vi "CAN 6 SPARK MAX Drivetrain Config.vi"() -> (14 "SPARK MAX Ref":T1={"FrontLeftMaster"={"DeviceStatus"={"status"=FALSE, "code"=0, "source"=""}, "Type"=enum."PWM", "PWM"={"PWM Channel"=enum."PWM 1", "DeadBand"={"Name"="", "maxPositivePwm"=0, "minPositivePwm"=0, "centerPwm"=0, "maxNegativePwm"=0, "minNegativePwm"=0, "angularRange"=0}}, "CAN"={"Device Number"=0, "SetOutput VI Ref"=variant(enum8{"Percent VBus", "Current", "Speed", "Position", "Voltage"} enum."Percent VBus"), "GetOutput VI Ref"=variant(refnum<k1> refnum), "Enable VI Ref"=variant(dbl 12.0), "Disable VI Ref"=variant(enum8{"Percent VBus", "Speed", "Position", "Slave", "Unchanged / Invalid", "Voltage Compensation", "Current", "Motion Profile"} enum."Percent VBus"), "Data"=variant}, "Invert"=FALSE, "DIO PWM"={"PWM \"Enable\" Channel"=enum."Invalid", "DIOChannel"=enum."Invalid", "PWM Rate"=0.0}}, "FrontLeftSlave1"={"DeviceStatus"={"status"=FALSE, "code"=0, "source"=""}, "Type"=enum."PWM", "PWM"={"PWM Channel"=enum."PWM 1", "DeadBand"={"Name"="", "maxPositivePwm"=0, "minPositivePwm"=0, "centerPwm"=0, "maxNegativePwm"=0, "minNegativePwm"=0, "angularRange"=0}}, "CAN"={"Device Number"=0, "SetOutput VI Ref"=variant(enum8{"Percent VBus", "Current", "Speed", "Position", "Voltage"} enum."Percent VBus"), "GetOutput VI Ref"=variant(refnum<k1> refnum), "Enable VI Ref"=variant(dbl 12.0), "Disable VI Ref"=variant(enum8{"Percent VBus", "Speed", "Position", "Slave", "Unchanged / Invalid", "Voltage Compensation", "Current", "Motion Profile"} enum."Percent VBus"), "Data"=variant}, "Invert"=FALSE, "DIO PWM"={"PWM \"Enable\" Channel"=enum."Invalid", "DIOChannel"=enum."Invalid", "PWM Rate"=0.0}}, "FrontLeftSlave2"={"DeviceStatus"={"status"=FALSE, "code"=0, "source"=""}, "Type"=enum."PWM", "PWM"={"PWM Channel"=enum."PWM 1", "DeadBand"={"Name"="", "maxPositivePwm"=0, "minPositivePwm"=0, "centerPwm"=0, "maxNegativePwm"=0, "minNegativePwm"=0, "angularRange"=0}}, "CAN"={"Device Number"=0, "SetOutput VI Ref"=variant(enum8{"Percent VBus", "Current", "Speed", "Position", "Voltage"} enum."Percent VBus"), "GetOutput VI Ref"=variant(refnum<k1> refnum), "Enable VI Ref"=variant(dbl 12.0), "Disable VI Ref"=variant(enum8{"Percent VBus", "Speed", "Position", "Slave", "Unchanged / Invalid", "Voltage Compensation", "Current", "Motion Profile"} enum."Percent VBus"), "Data"=variant}, "Invert"=FALSE, "DIO PWM"={"PWM \"Enable\" Channel"=enum."Invalid", "DIOChannel"=enum."Invalid", "PWM Rate"=0.0}}, "FrontRightMaster"={"DeviceStatus"={"status"=FALSE, "code"=0, "source"=""}, "Type"=enum."PWM", "PWM"={"PWM Channel"=enum."PWM 1", "DeadBand"={"Name"="", "maxPositivePwm"=0, "minPositivePwm"=0, "centerPwm"=0, "maxNegativePwm"=0, "minNegativePwm"=0, "angularRange"=0}}, "CAN"={"Device Number"=0, "SetOutput VI Ref"=variant(enum8{"Percent VBus", "Current", "Speed", "Position", "Voltage"} enum."Percent VBus"), "GetOutput VI Ref"=variant(refnum<k1> refnum), "Enable VI Ref"=variant(dbl 12.0), "Disable VI Ref"=variant(enum8{"Percent VBus", "Speed", "Position", "Slave", "Unchanged / Invalid", "Voltage Compensation", "Current", "Motion Profile"} enum."Percent VBus"), "Data"=variant}, "Invert"=FALSE, "DIO PWM"={"PWM \"Enable\" Channel"=enum."Invalid", "DIOChannel"=enum."Invalid", "PWM Rate"=0.0}}, "FrontRightSlave1"={"DeviceStatus"={"status"=FALSE, "code"=0, "source"=""}, "Type"=enum."PWM", "PWM"={"PWM Channel"=enum."PWM 1", "DeadBand"={"Name"="", "maxPositivePwm"=0, "minPositivePwm"=0, "centerPwm"=0, "maxNegativePwm"=0, "minNegativePwm"=0, "angularRange"=0}}, "CAN"={"Device Number"=0, "SetOutput VI Ref"=variant(enum8{"Percent VBus", "Current", "Speed", "Position", "Voltage"} enum."Percent VBus"), "GetOutput VI Ref"=variant(refnum<k1> refnum), "Enable VI Ref"=variant(dbl 12.0), "Disable VI Ref"=variant(enum8{"Percent VBus", "Speed", "Position", "Slave", "Unchanged / Invalid", "Voltage Compensation", "Current", "Motion Profile"} enum."Percent VBus"), "Data"=variant}, "Invert"=FALSE, "DIO PWM"={"PWM \"Enable\" Channel"=enum."Invalid", "DIOChannel"=enum."Invalid", "PWM Rate"=0.0}}, "FrontRightSlave2"={"DeviceStatus"={"status"=FALSE, "code"=0, "source"=""}, "Type"=enum."PWM", "PWM"={"PWM Channel"=enum."PWM 1", "DeadBand"={"Name"="", "maxPositivePwm"=0, "minPositivePwm"=0, "centerPwm"=0, "maxNegativePwm"=0, "minNegativePwm"=0, "angularRange"=0}}, "CAN"={"Device Number"=0, "SetOutput VI Ref"=variant(enum8{"Percent VBus", "Current", "Speed", "Position", "Voltage"} enum."Percent VBus"), "GetOutput VI Ref"=variant(refnum<k1> refnum), "Enable VI Ref"=variant(dbl 12.0), "Disable VI Ref"=variant(enum8{"Percent VBus", "Speed", "Position", "Slave", "Unchanged / Invalid", "Voltage Compensation", "Current", "Motion Profile"} enum."Percent VBus"), "Data"=variant}, "Invert"=FALSE, "DIO PWM"={"PWM \"Enable\" Channel"=enum."Invalid", "DIOChannel"=enum."Invalid", "PWM Rate"=0.0}}})   [LabVIEW 2018]
uses:
  SPARKMAX6Motor.ctl
  <vilib>/Rock Robotics/WPI/MotorControl/WPI_MotorControlDeviceRef.ctl
  <vilib>/Rock Robotics/WPI/MotorControl/WPI_MotorControlType.ctl
  <vilib>/Rock Robotics/SystemInterfaces/DIO/FPGA_DIOPWMChannel.ctl
  <vilib>/Rock Robotics/WPI/PWM/WPI_PWMDeadband.ctl
  <vilib>/Rock Robotics/SystemInterfaces/DIO/FPGA_DIOChannel.ctl
  <vilib>/Rock Robotics/WPI/ThirdParty/REV Robotics/SPARK MAX/Typedef/Spark MAX Status Frames.ctl
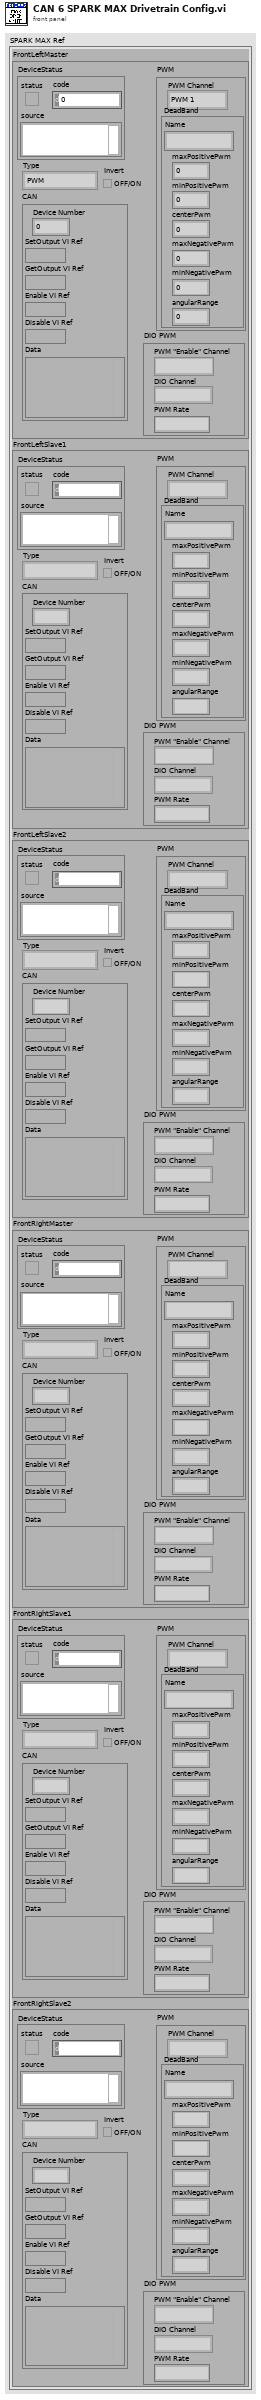
[diagram p1: front panel]
types:
  T1 = typedef "SPARKMAX6Motor.ctl" = cluster{"FrontLeftMaster":T2, "FrontLeftSlave1":T2, "FrontLeftSlave2":T2, "FrontRightMaster":T2, "FrontRightSlave1":T2, "FrontRightSlave2":T2}
  T2 = typedef "WPI_MotorControlDeviceRef.ctl" = cluster{"DeviceStatus":errorcluster, "Type":T3, "PWM":cluster{"PWM Channel":T4, "DeadBand":T5}, "CAN":cluster{"Device Number":u8, "SetOutput VI Ref":variant, "GetOutput VI Ref":variant, "Enable VI Ref":variant, "Disable VI Ref":variant, "Data":variant}, "Invert":bool, "DIO PWM":cluster{"PWM \"Enable\" Channel":T4, "DIOChannel":T6, "PWM Rate":dbl}}
  T3 = typedef "WPI_MotorControlType.ctl" = enum16{"PWM", "CAN", "DIO PWM"}
  T4 = typedef "FPGA_DIOPWMChannel.ctl" = enum8{"PWM 0", "PWM 1", "PWM 2", "PWM 3", "PWM 4", "PWM 5", "PWM 6", "PWM 7", "PWM 8", "PWM 9", "PWM MXP 0", "PWM MXP 1", "PWM MXP 2", "PWM MXP 3", "PWM MXP 4", "PWM MXP 5", "PWM MXP 6", "PWM MXP 7", "PWM MXP 8", "PWM MXP 9", "Invalid"}
  T5 = typedef "WPI_PWMDeadband.ctl" = cluster{"Name":string, "maxPositivePwm":i32, "minPositivePwm":i32, "centerPwm":i32, "maxNegativePwm":i32, "minNegativePwm":i32, "angularRange":u16}
  T6 = typedef "FPGA_DIOChannel.ctl" = enum8{"DIO 0", "DIO 1", "DIO 2", "DIO 3", "DIO 4", "DIO 5", "DIO 6", "DIO 7", "DIO 8", "DIO 9", "DIO MXP 0", "DIO MXP 1", "DIO MXP 2", "DIO MXP 3", "DIO MXP 4", "DIO MXP 5", "DIO MXP 6", "DIO MXP 7", "DIO MXP 8", "DIO MXP 9", "DIO MXP 10", "DIO MXP 11", "DIO MXP 12", "DIO MXP 13", "DIO MXP 14", "DIO MXP 15", "SPI Port CS1", "SPI Port CS2", "SPI Port CS3", "SPI Port MISO", "SPI Port MOSI", "Invalid"}
  T7 = typedef "Spark MAX Status Frames.ctl" = enum16{"Status 0", "Status 1", "Status 2"}
  T8 = cluster{"P Gain":dbl, "I Gain":dbl, "D Gain":dbl, "F Gain":dbl, "I Zone":dbl, "Min Output":dbl, "Max Output":dbl}
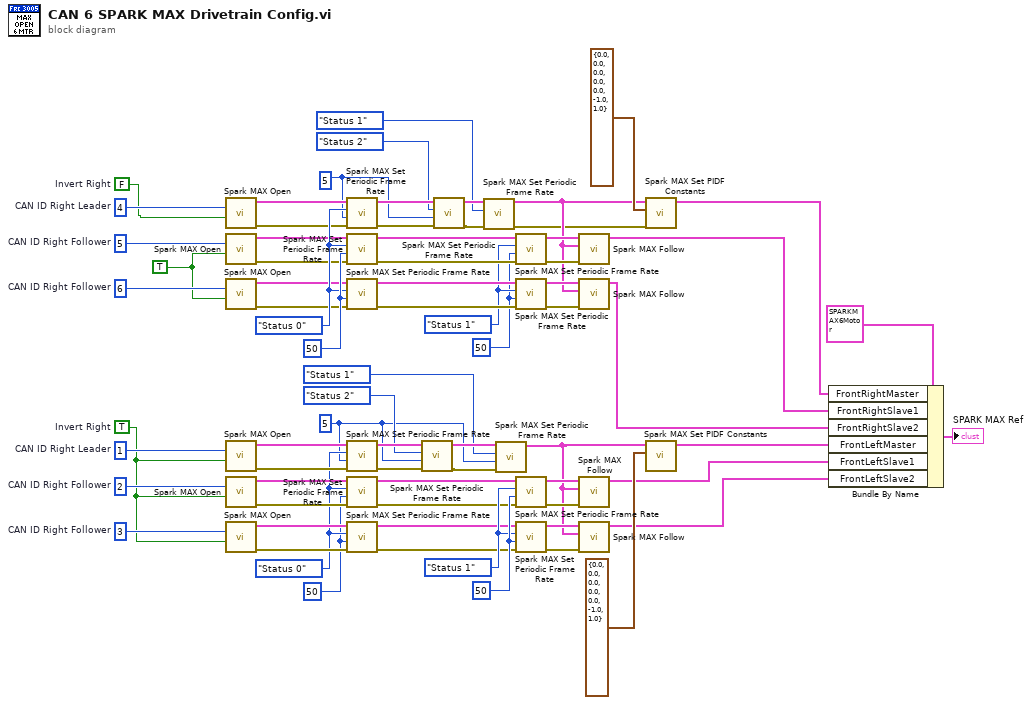
[diagram p0: block diagram]
diagram:
  w1 = TRUE
  w40 = u16 50 ("Frame rate (ms)")
  w41 = Spark_MAX_Status_Frames."Status 1" ("Frame")
  w39 = u16 50 ("Frame rate (ms)")
  w16 = u16 5 ("Frame rate (ms)")
  w38 = Spark_MAX_Status_Frames."Status 0" ("Frame")
  w31 = u8 6  # CAN ID Right Follower
  w3 = FALSE  # Invert Right
  w29 = u8 4  # CAN ID Right Leader
  w30 = u8 5  # CAN ID Right Follower
  w61 = u16 50 ("Frame rate (ms)")
  w60 = Spark_MAX_Status_Frames."Status 1" ("Frame")
  w62 = u16 50 ("Frame rate (ms)")
  w4 = u16 5 ("Frame rate (ms)")
  w63 = Spark_MAX_Status_Frames."Status 0" ("Frame")
  w70 = u8 3  # CAN ID Right Follower
  w2 = TRUE  # Invert Right
  w72 = u8 1  # CAN ID Right Leader
  w71 = u8 2  # CAN ID Right Follower
  n1 = call <vilib>:"Spark MAX Open.vi"("Invert"=w3, "Device Number"=w29) -> ("error out"=w37:errorcluster, "MotorControlDeviceRef"=w36:T2)  [unwired: 8 in]
  n2 = call <vilib>:"Spark MAX Open.vi"("Invert"=w1, "Device Number"=w30) -> ("error out"=w34:errorcluster, "MotorControlDeviceRef"=w35:T2)  [unwired: 8 in]
  n3 = call <vilib>:"Spark MAX Open.vi"("Invert"=w1, "Device Number"=w31) -> ("error out"=w32:errorcluster, "MotorControlDeviceRef"=w33:T2)  [unwired: 8 in]
  n4 = call <vilib>:"Spark MAX Open.vi"("Invert"=w2, "Device Number"=w72) -> ("error out"=w64:errorcluster, "MotorControlDeviceRef"=w65:T2)  [unwired: 8 in]
  n5 = call <vilib>:"Spark MAX Open.vi"("Invert"=w2, "Device Number"=w71) -> ("error out"=w67:errorcluster, "MotorControlDeviceRef"=w66:T2)  [unwired: 8 in]
  n6 = call <vilib>:"Spark MAX Open.vi"("Invert"=w2, "Device Number"=w70) -> ("error out"=w69:errorcluster, "MotorControlDeviceRef"=w68:T2)  [unwired: 8 in]
  n7 = call <vilib>:"Spark MAX Set Periodic Frame Rate.vi"("error in"=w37, "Frame rate (ms)"=w16, "Frame"=w38, "MotorControlDeviceRef"=w36) -> ("error out"=w20:errorcluster, "MotorControlDeviceRef"=w19:T2)  [unwired: 6 in]
  n8 = call <vilib>:"Spark MAX Set Periodic Frame Rate.vi"("error in"=w34, "Frame rate (ms)"=w39, "Frame"=w38, "MotorControlDeviceRef"=w35) -> ("error out"=w45:errorcluster, "MotorControlDeviceRef"=w42:T2)  [unwired: 6 in]
  n9 = call <vilib>:"Spark MAX Set Periodic Frame Rate.vi"("error in"=w32, "Frame rate (ms)"=w39, "Frame"=w38, "MotorControlDeviceRef"=w33) -> ("error out"=w44:errorcluster, "MotorControlDeviceRef"=w43:T2)  [unwired: 6 in]
  n10 = call <vilib>:"Spark MAX Set Periodic Frame Rate.vi"("error in"=w64, "Frame rate (ms)"=w4, "Frame"=w63, "MotorControlDeviceRef"=w65) -> ("error out"=w8:errorcluster, "MotorControlDeviceRef"=w9:T2)  [unwired: 6 in]
  n11 = call <vilib>:"Spark MAX Set Periodic Frame Rate.vi"("error in"=w67, "Frame rate (ms)"=w62, "Frame"=w63, "MotorControlDeviceRef"=w66) -> ("error out"=w56:errorcluster, "MotorControlDeviceRef"=w59:T2)  [unwired: 6 in]
  n12 = call <vilib>:"Spark MAX Set Periodic Frame Rate.vi"("error in"=w69, "Frame rate (ms)"=w62, "Frame"=w63, "MotorControlDeviceRef"=w68) -> ("error out"=w57:errorcluster, "MotorControlDeviceRef"=w58:T2)  [unwired: 6 in]
  n13 = call <vilib>:"Spark MAX Set Periodic Frame Rate.vi"("error in"=w8, "Frame rate (ms)"=w4, "Frame"=Spark_MAX_Status_Frames."Status 2", "MotorControlDeviceRef"=w9) -> ("error out"=w11:errorcluster, "MotorControlDeviceRef"=w10:T2)  [unwired: 6 in]
  n14 = call <vilib>:"Spark MAX Set Periodic Frame Rate.vi"("error in"=w20, "Frame rate (ms)"=w16, "Frame"=Spark_MAX_Status_Frames."Status 2", "MotorControlDeviceRef"=w19) -> ("error out"=w17:errorcluster, "MotorControlDeviceRef"=w18:T2)  [unwired: 6 in]
  n15 = call <vilib>:"Spark MAX Set Periodic Frame Rate.vi"("error in"=w17, "Frame"=Spark_MAX_Status_Frames."Status 1", "MotorControlDeviceRef"=w18) -> ("error out"=w12:errorcluster, "MotorControlDeviceRef"=w13:T2)  [unwired: 7 in]
  n16 = call <vilib>:"Spark MAX Set Periodic Frame Rate.vi"("error in"=w11, "Frame rate (ms)"=w4, "Frame"=Spark_MAX_Status_Frames."Status 1", "MotorControlDeviceRef"=w10) -> ("MotorControlDeviceRef"=w7:T2)  [unwired: 6 in, 1 out]
  n17 = call <vilib>:"Spark MAX Set Periodic Frame Rate.vi"("error in"=w45, "Frame rate (ms)"=w40, "Frame"=w41, "MotorControlDeviceRef"=w42) -> ("error out"=w47:errorcluster, "MotorControlDeviceRef"=w46:T2)  [unwired: 6 in]
  n18 = call <vilib>:"Spark MAX Set Periodic Frame Rate.vi"("error in"=w44, "Frame rate (ms)"=w40, "Frame"=w41, "MotorControlDeviceRef"=w43) -> ("error out"=w48:errorcluster, "MotorControlDeviceRef"=w49:T2)  [unwired: 6 in]
  n19 = call <vilib>:"Spark MAX Set Periodic Frame Rate.vi"("error in"=w56, "Frame rate (ms)"=w61, "Frame"=w60, "MotorControlDeviceRef"=w59) -> ("error out"=w54:errorcluster, "MotorControlDeviceRef"=w55:T2)  [unwired: 6 in]
  n20 = call <vilib>:"Spark MAX Set Periodic Frame Rate.vi"("error in"=w57, "Frame rate (ms)"=w61, "Frame"=w60, "MotorControlDeviceRef"=w58) -> ("error out"=w53:errorcluster, "MotorControlDeviceRef"=w52:T2)  [unwired: 6 in]
  n21 = call <vilib>:"Spark MAX Follow.vi"("error in (no error)"=w47, "Master Controller"=w13, "MotorControlDeviceRef"=w46) -> ("MotorControlDeviceRef"=w22:T2)  [unwired: 7 in, 1 out]
  n22 = call <vilib>:"Spark MAX Follow.vi"("error in (no error)"=w48, "Master Controller"=w13, "MotorControlDeviceRef"=w49) -> ("MotorControlDeviceRef"=w23:T2)  [unwired: 7 in, 1 out]
  n23 = call <vilib>:"Spark MAX Follow.vi"("error in (no error)"=w54, "Master Controller"=w7, "MotorControlDeviceRef"=w55) -> ("MotorControlDeviceRef"=w25:T2)  [unwired: 7 in, 1 out]
  n24 = call <vilib>:"Spark MAX Follow.vi"("error in (no error)"=w53, "Master Controller"=w7, "MotorControlDeviceRef"=w52) -> ("MotorControlDeviceRef"=w24:T2)  [unwired: 7 in, 1 out]
  n25 = call <vilib>:"Spark MAX Set PIDF Constants.vi"("error in"=w12, "PID Constants"=T8 {"P Gain"=0.0, "I Gain"=0.0, "D Gain"=0.0, "F Gain"=0.0, "I Zone"=0.0, "Min Output"=-1.0, "Max Output"=1.0}, "MotorControlDeviceRef"=w13) -> ("MotorControlDeviceRef"=w27:T2)  [unwired: 7 in, 1 out]
  n26 = call <vilib>:"Spark MAX Set PIDF Constants.vi"("PID Constants"=T8 {"P Gain"=0.0, "I Gain"=0.0, "D Gain"=0.0, "F Gain"=0.0, "I Zone"=0.0, "Min Output"=-1.0, "Max Output"=1.0}, "MotorControlDeviceRef"=w7) -> ("MotorControlDeviceRef"=w26:T2)  [unwired: 8 in, 1 out]
  n27 = Bundle By Name(cluster=T1 {"FrontLeftMaster"={"DeviceStatus"={"status"=FALSE, "code"=0, "source"=""}, "Type"=enum."PWM", "PWM"={"PWM Channel"=enum."PWM 1", "DeadBand"={"Name"="", "maxPositivePwm"=0, "minPositivePwm"=0, "centerPwm"=0, "maxNegativePwm"=0, "minNegativePwm"=0, "angularRange"=0}}, "CAN"={"Device Number"=0, "SetOutput VI Ref"=variant(enum8{"Percent VBus", "Current", "Speed", "Position", "Voltage"} enum."Percent VBus"), "GetOutput VI Ref"=variant(refnum<k1> refnum), "Enable VI Ref"=variant(dbl 12.0), "Disable VI Ref"=variant(enum8{"Percent VBus", "Speed", "Position", "Slave", "Unchanged / Invalid", "Voltage Compensation", "Current", "Motion Profile"} enum."Percent VBus"), "Data"=variant}, "Invert"=FALSE, "DIO PWM"={"PWM \"Enable\" Channel"=enum."Invalid", "DIOChannel"=enum."Invalid", "PWM Rate"=0.0}}, "FrontLeftSlave1"={"DeviceStatus"={"status"=FALSE, "code"=0, "source"=""}, "Type"=enum."PWM", "PWM"={"PWM Channel"=enum."PWM 1", "DeadBand"={"Name"="", "maxPositivePwm"=0, "minPositivePwm"=0, "centerPwm"=0, "maxNegativePwm"=0, "minNegativePwm"=0, "angularRange"=0}}, "CAN"={"Device Number"=0, "SetOutput VI Ref"=variant(enum8{"Percent VBus", "Current", "Speed", "Position", "Voltage"} enum."Percent VBus"), "GetOutput VI Ref"=variant(refnum<k1> refnum), "Enable VI Ref"=variant(dbl 12.0), "Disable VI Ref"=variant(enum8{"Percent VBus", "Speed", "Position", "Slave", "Unchanged / Invalid", "Voltage Compensation", "Current", "Motion Profile"} enum."Percent VBus"), "Data"=variant}, "Invert"=FALSE, "DIO PWM"={"PWM \"Enable\" Channel"=enum."Invalid", "DIOChannel"=enum."Invalid", "PWM Rate"=0.0}}, "FrontLeftSlave2"={"DeviceStatus"={"status"=FALSE, "code"=0, "source"=""}, "Type"=enum."PWM", "PWM"={"PWM Channel"=enum."PWM 1", "DeadBand"={"Name"="", "maxPositivePwm"=0, "minPositivePwm"=0, "centerPwm"=0, "maxNegativePwm"=0, "minNegativePwm"=0, "angularRange"=0}}, "CAN"={"Device Number"=0, "SetOutput VI Ref"=variant(enum8{"Percent VBus", "Current", "Speed", "Position", "Voltage"} enum."Percent VBus"), "GetOutput VI Ref"=variant(refnum<k1> refnum), "Enable VI Ref"=variant(dbl 12.0), "Disable VI Ref"=variant(enum8{"Percent VBus", "Speed", "Position", "Slave", "Unchanged / Invalid", "Voltage Compensation", "Current", "Motion Profile"} enum."Percent VBus"), "Data"=variant}, "Invert"=FALSE, "DIO PWM"={"PWM \"Enable\" Channel"=enum."Invalid", "DIOChannel"=enum."Invalid", "PWM Rate"=0.0}}, "FrontRightMaster"={"DeviceStatus"={"status"=FALSE, "code"=0, "source"=""}, "Type"=enum."PWM", "PWM"={"PWM Channel"=enum."PWM 1", "DeadBand"={"Name"="", "maxPositivePwm"=0, "minPositivePwm"=0, "centerPwm"=0, "maxNegativePwm"=0, "minNegativePwm"=0, "angularRange"=0}}, "CAN"={"Device Number"=0, "SetOutput VI Ref"=variant(enum8{"Percent VBus", "Current", "Speed", "Position", "Voltage"} enum."Percent VBus"), "GetOutput VI Ref"=variant(refnum<k1> refnum), "Enable VI Ref"=variant(dbl 12.0), "Disable VI Ref"=variant(enum8{"Percent VBus", "Speed", "Position", "Slave", "Unchanged / Invalid", "Voltage Compensation", "Current", "Motion Profile"} enum."Percent VBus"), "Data"=variant}, "Invert"=FALSE, "DIO PWM"={"PWM \"Enable\" Channel"=enum."Invalid", "DIOChannel"=enum."Invalid", "PWM Rate"=0.0}}, "FrontRightSlave1"={"DeviceStatus"={"status"=FALSE, "code"=0, "source"=""}, "Type"=enum."PWM", "PWM"={"PWM Channel"=enum."PWM 1", "DeadBand"={"Name"="", "maxPositivePwm"=0, "minPositivePwm"=0, "centerPwm"=0, "maxNegativePwm"=0, "minNegativePwm"=0, "angularRange"=0}}, "CAN"={"Device Number"=0, "SetOutput VI Ref"=variant(enum8{"Percent VBus", "Current", "Speed", "Position", "Voltage"} enum."Percent VBus"), "GetOutput VI Ref"=variant(refnum<k1> refnum), "Enable VI Ref"=variant(dbl 12.0), "Disable VI Ref"=variant(enum8{"Percent VBus", "Speed", "Position", "Slave", "Unchanged / Invalid", "Voltage Compensation", "Current", "Motion Profile"} enum."Percent VBus"), "Data"=variant}, "Invert"=FALSE, "DIO PWM"={"PWM \"Enable\" Channel"=enum."Invalid", "DIOChannel"=enum."Invalid", "PWM Rate"=0.0}}, "FrontRightSlave2"={"DeviceStatus"={"status"=FALSE, "code"=0, "source"=""}, "Type"=enum."PWM", "PWM"={"PWM Channel"=enum."PWM 1", "DeadBand"={"Name"="", "maxPositivePwm"=0, "minPositivePwm"=0, "centerPwm"=0, "maxNegativePwm"=0, "minNegativePwm"=0, "angularRange"=0}}, "CAN"={"Device Number"=0, "SetOutput VI Ref"=variant(enum8{"Percent VBus", "Current", "Speed", "Position", "Voltage"} enum."Percent VBus"), "GetOutput VI Ref"=variant(refnum<k1> refnum), "Enable VI Ref"=variant(dbl 12.0), "Disable VI Ref"=variant(enum8{"Percent VBus", "Speed", "Position", "Slave", "Unchanged / Invalid", "Voltage Compensation", "Current", "Motion Profile"} enum."Percent VBus"), "Data"=variant}, "Invert"=FALSE, "DIO PWM"={"PWM \"Enable\" Channel"=enum."Invalid", "DIOChannel"=enum."Invalid", "PWM Rate"=0.0}}} ("TalonSRX6Motor"), "FrontRightMaster"=w27, "FrontRightSlave1"=w22, "FrontRightSlave2"=w23, "FrontLeftMaster"=w26, "FrontLeftSlave1"=w25, "FrontLeftSlave2"=w24) -> (→"SPARK MAX Ref":T1)
